vi "write_params.vi"(8 "error in (no error)":errorcluster, 10 "params":T1={"min_samples"=5.0, "max_eps"=inf, "metric"="euclidean", "p"=2.0, "cluster_method"="xi", "eps"={"eps_type"="None", "eps_float"=0.0}, "xi"=0.05, "predecessor_correction"=TRUE, "min_cluster_size"={"min_cluster_size_type"="None", "min_cluster_size_int"=1.0, "min_cluster_size_float"=0.0}, "algorithm"="auto", "leaf_size"=30.0, "n_jobs"=1.0}, 11 "OPTICS in":refnum<class "OPTICS.lvclass">) -> (0 "error out":errorcluster, 3 "OPTICS out":refnum<class "OPTICS.lvclass">)   [LabVIEW 2020, in "OPTICS.lvclass"]
uses:
  OPTICS.lvclass
  Controls/optics_params.ctl
  OPTICS.lvclass/OPTICS.ctl
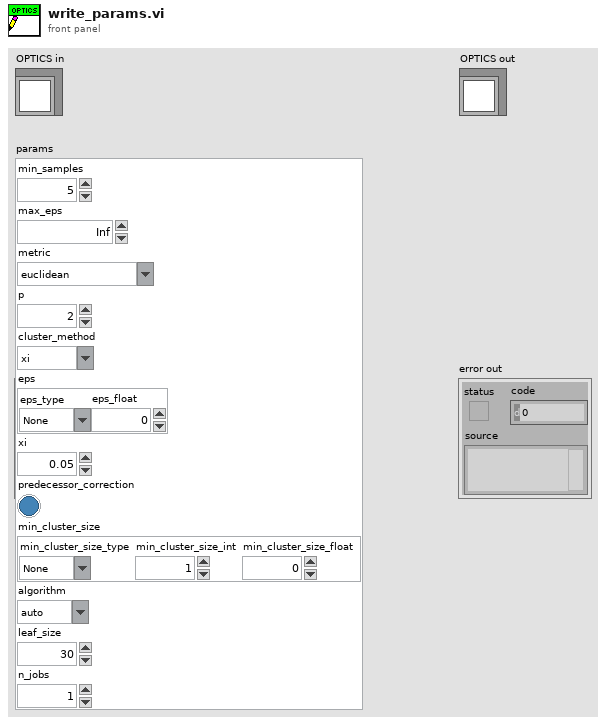
[diagram p1: front panel]
types:
  T1 = typedef "optics_params.ctl" = cluster{"min_samples":dbl, "max_eps":dbl, "metric":string, "p":dbl, "cluster_method":string, "eps":cluster{"eps_type":string, "eps_float":dbl}, "xi":dbl, "predecessor_correction":bool, "min_cluster_size":cluster{"min_cluster_size_type":string, "min_cluster_size_int":dbl, "min_cluster_size_float":dbl}, "algorithm":string, "leaf_size":dbl, "n_jobs":dbl}
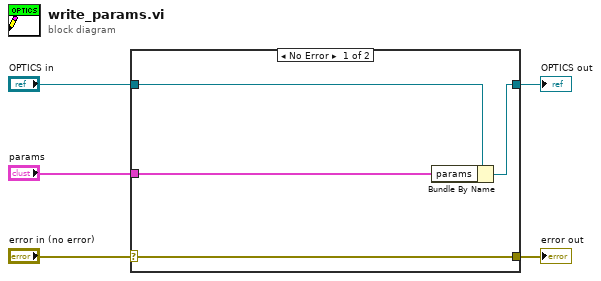
[diagram p0: block diagram]
diagram:
  n1 = case shown="No Error" "error in (no error)" {
    selector: "error in (no error)" -> [w9 w10]
    tunnel: [w9 w10] -> w4
    tunnel: [w7 w11] -> w2
    tunnel: "OPTICS in" -> [w8 w11]
    tunnel: "params" -> [w6 _]
    frame No Error {
      n2 = Bundle By Name(cluster=w8, "params"=w6) -> (w7:refnum<class "OPTICS.lvclass">)
    }
    frame Error {
    }
  }
  "error out" <- w4
  "OPTICS out" <- w2
